vi "Hall Effect Current Sensor Conversion.vi"(2 "Hall Effect Sensor Voltage (V)":dbl) -> (7 "Hall Effect Sensor Current (A)":dbl)   [LabVIEW 2017]
panel:
  # "This is specific for the ACS722LLCTR-20AB-T Hall-Effect current sensor"
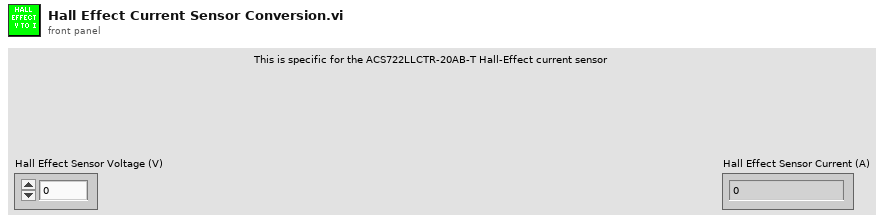
[diagram p1: front panel]
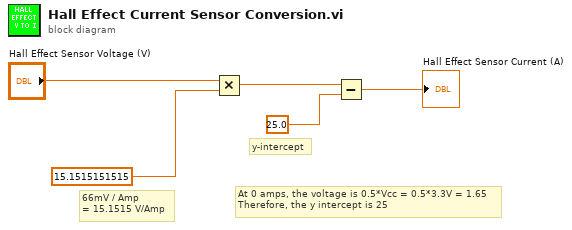
[diagram p0: block diagram]
diagram:
  # "y-intercept"
  # "At 0 amps, the voltage is 0.5*Vcc = 0.5*3.3V = 1.65\nTherefore, the y intercept is 25"
  # "66mV / Amp\n= 15.1515 V/Amp"
  n1 = Multiply(x="Hall Effect Sensor Voltage (V)", y=15.1515151515) -> (x*y=w2:dbl)
  n2 = Subtract(x=w2, y=25.0) -> (x-y=→"Hall Effect Sensor Current (A)":dbl)
